vi "Sample_Data_Compute.vi"(8 "Data Array 2":dbl[][](array[numeric]), 11 "Data Array 1":dbl[][](array[numeric])) -> (0 "Cam2_Stats":cluster{"Mean_Area":i32, "Img_Count":u32} caption="Camera 2", 1 "Cam1_Stats":cluster{"Mean_Area":i32, "Img_Count":u32} caption="Camera 1", 2 "Arear mean":dbl format="%0.2f", 3 "output cluster":T1)   [LabVIEW 2024]
uses:
  <vilib>/Analysis/NI_AALBase.lvlib
panel:
  in  "Data Cluster":T1
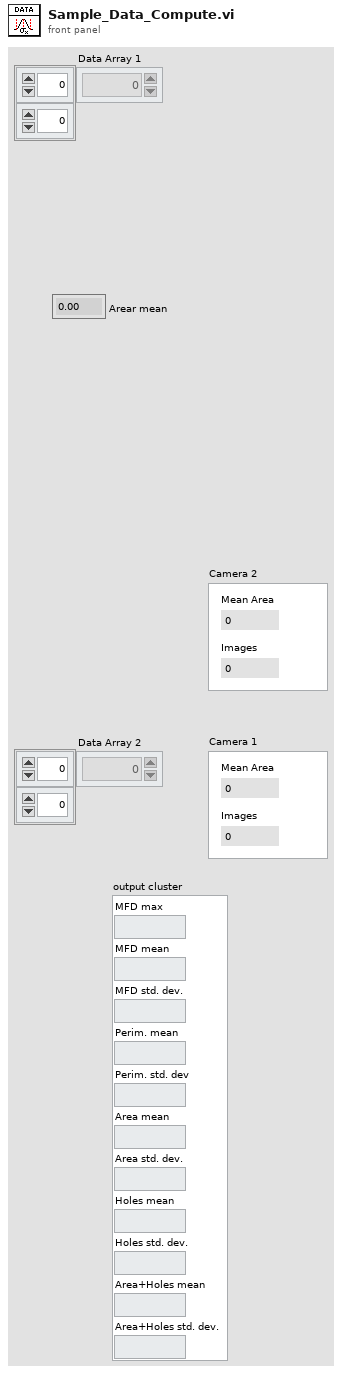
[diagram p1: front panel]
types:
  T1 = cluster{"MFD max":string, "MFD mean":string, "MFD std. dev.":string, "Perim. mean":string, "Perim. std. dev":string, "Area mean":string, "Area std. dev.":string, "Holes mean":string, "Holes std. dev.":string, "Area+Holes mean":string, "Area+Holes std. dev.":string}
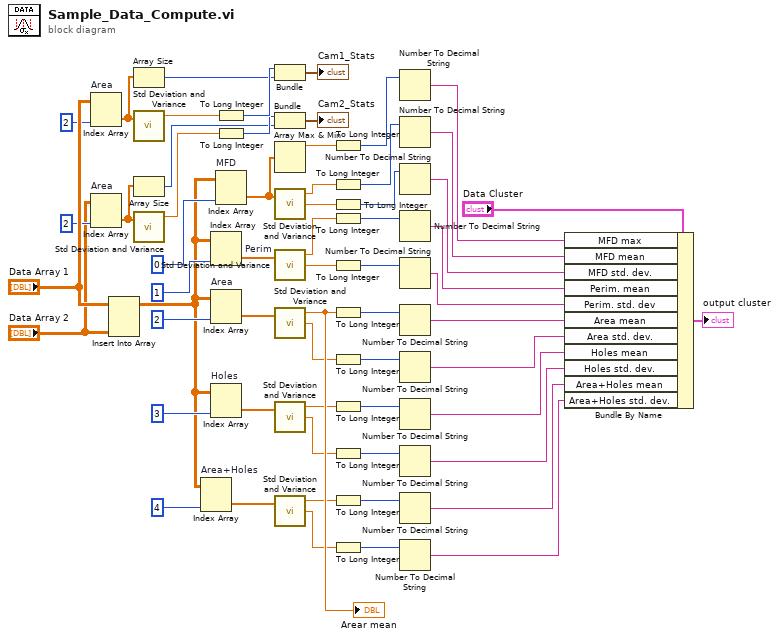
[diagram p0: block diagram]
diagram:
  n1 = Index Array "Area"(array="Data Array 1", index (col)=2 ("disabled index (col)")) -> (element=w9:dbl[])  [unwired: 1 in]
  n2 = Index Array "Area"(array="Data Array 2", index (col)=2 ("disabled index (col)")) -> (element=w8:dbl[])  [unwired: 1 in]
  n3 = Insert Into Array(array="Data Array 1", new element="Data Array 2") -> (w21:dbl[][])  [unwired: 2 in]
  n4 = Array Size(array=w9) -> (size(s)=w6:i32)
  n5 = call <vilib>:"Std Deviation and Variance.vi"("X"=w9) -> ("mean"=w15:dbl)  [unwired: 1 in, 2 out]
  n6 = Array Size(array=w8) -> (size(s)=w4:i32)
  n7 = call <vilib>:"Std Deviation and Variance.vi"("X"=w8) -> ("mean"=w11:dbl)  [unwired: 1 in, 2 out]
  n8 = Index Array "Area+Holes"(array=w21, index (col)=4 ("disabled index (col)")) -> (element=w16:dbl[])  [unwired: 1 in]
  n9 = Index Array "Perim"(array=w21, index (col)=1 ("disabled index (col)")) -> (element=w19:dbl[])  [unwired: 1 in]
  n10 = Index Array "Area"(array=w21, index (col)=2 ("disabled index (col)")) -> (element=w18:dbl[])  [unwired: 1 in]
  n11 = Index Array "Holes"(array=w21, index (col)=3 ("disabled index (col)")) -> (element=w17:dbl[])  [unwired: 1 in]
  n12 = To Long Integer(number=w15) -> (32bit integer=w7:i32)
  n13 = To Long Integer(number=w11) -> (32bit integer=w5:i32)
  n14 = Index Array "MFD"(array=w21, index (col)=0 ("disabled index (col)")) -> (element=w20:dbl[])  [unwired: 1 in]
  n15 = Bundle(w7, w6) -> (→"Cam1_Stats":cluster{i32, i32})  [unwired: 1 in]
  n16 = Bundle(w5, w4) -> (→"Cam2_Stats":cluster{i32, i32})  [unwired: 1 in]
  n17 = Array Max & Min(array=w20) -> (max value=w60:dbl)  [unwired: 3 out]
  n18 = call <vilib>:"Std Deviation and Variance.vi"("X"=w20) -> ("mean"=w31:dbl, "standard deviation"=w30:dbl)  [unwired: 1 in, 1 out]
  n19 = call <vilib>:"Std Deviation and Variance.vi"("X"=w19) -> ("mean"=w53:dbl, "standard deviation"=w50:dbl)  [unwired: 1 in, 1 out]
  n20 = call <vilib>:"Std Deviation and Variance.vi"("X"=w18) -> ("mean"=w48:dbl, "standard deviation"=w45:dbl)  [unwired: 1 in, 1 out]
  "Arear mean" <- w48
  n21 = call <vilib>:"Std Deviation and Variance.vi"("X"=w17) -> ("mean"=w43:dbl, "standard deviation"=w39:dbl)  [unwired: 1 in, 1 out]
  n22 = call <vilib>:"Std Deviation and Variance.vi"("X"=w16) -> ("mean"=w36:dbl, "standard deviation"=w35:dbl)  [unwired: 1 in, 1 out]
  n23 = To Long Integer(number=w60) -> (32bit integer=w59:i32)
  n24 = To Long Integer(number=w31) -> (32bit integer=w33:i32)
  n25 = To Long Integer(number=w30) -> (32bit integer=w32:i32)
  n26 = To Long Integer(number=w53) -> (32bit integer=w58:i32)
  n27 = To Long Integer(number=w50) -> (32bit integer=w57:i32)
  n28 = To Long Integer(number=w48) -> (32bit integer=w56:i32)
  n29 = To Long Integer(number=w45) -> (32bit integer=w55:i32)
  n30 = To Long Integer(number=w43) -> (32bit integer=w54:i32)
  n31 = To Long Integer(number=w39) -> (32bit integer=w42:i32)
  n32 = To Long Integer(number=w36) -> (32bit integer=w41:i32)
  n33 = To Long Integer(number=w35) -> (32bit integer=w40:i32)
  n34 = Number To Decimal String(number=w59) -> (decimal integer string=w28:string)  [unwired: 1 in]
  n35 = Number To Decimal String(number=w33) -> (decimal integer string=w29:string)  [unwired: 1 in]
  n36 = Number To Decimal String(number=w32) -> (decimal integer string=w27:string)  [unwired: 1 in]
  n37 = Number To Decimal String(number=w58) -> (decimal integer string=w52:string)  [unwired: 1 in]
  n38 = Number To Decimal String(number=w57) -> (decimal integer string=w49:string)  [unwired: 1 in]
  n39 = Number To Decimal String(number=w56) -> (decimal integer string=w47:string)  [unwired: 1 in]
  n40 = Number To Decimal String(number=w55) -> (decimal integer string=w46:string)  [unwired: 1 in]
  n41 = Number To Decimal String(number=w54) -> (decimal integer string=w44:string)  [unwired: 1 in]
  n42 = Number To Decimal String(number=w42) -> (decimal integer string=w38:string)  [unwired: 1 in]
  n43 = Number To Decimal String(number=w41) -> (decimal integer string=w37:string)  [unwired: 1 in]
  n44 = Number To Decimal String(number=w40) -> (decimal integer string=w34:string)  [unwired: 1 in]
  n45 = Bundle By Name(cluster="Data Cluster", "MFD max"=w28, "MFD mean"=w29, "MFD std. dev."=w27, "Perim. mean"=w52, "Perim. std. dev"=w49, "Area mean"=w47, "Area std. dev."=w46, "Holes mean"=w44, "Holes std. dev."=w38, "Area+Holes mean"=w37, "Area+Holes std. dev."=w34) -> (→"output cluster":T1)
